vi "picoCoAdd.vi"(8 "error in (no error)":errorcluster, 10 "Buffer In":i16[][](array[numeric])) -> (0 "error out":errorcluster, 2 "Waveform Out":dbl[](array[numeric]))   [LabVIEW 2011]
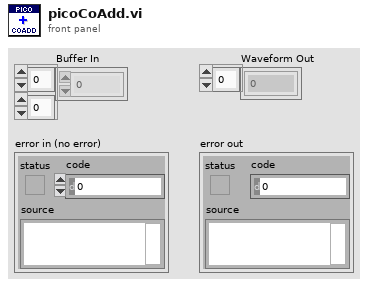
[diagram p1: front panel]
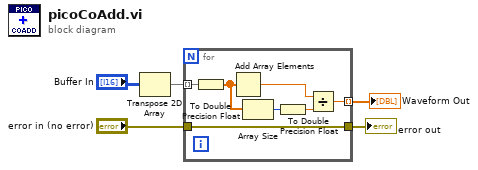
[diagram p0: block diagram]
diagram:
  n1 = Transpose 2D Array(2D array="Buffer In") -> (transposed array=w1:i16[][])
  n2 = for {
    tunnel: w1 -> [w8] mode=indexing
    tunnel: "error in (no error)" -> [w12]
    tunnel: [w12] -> w5
    tunnel: [w6] -> w3 mode=indexing
    n3 = To Double Precision Float(number=w8) -> (double precision float=w7:dbl[])
    n4 = Add Array Elements(numeric array=w7) -> (sum=w9:dbl)
    n5 = Array Size(array=w7) -> (size(s)=w11:i32)
    n6 = To Double Precision Float(number=w11) -> (double precision float=w10:dbl)
    n7 = Divide(x=w9, y=w10) -> (x/y=w6:dbl)
  }
  "error out" <- w5
  "Waveform Out" <- w3
